vi "LR-Spikes.vi"(5 "Test characteristics":T2, 7 "Spike detection settings":cluster{"Treshold [%]":i32}={"Treshold [%]"=10}, 8 "error in (no error)":errorcluster, 9 "Power in":dbl[](array[numeric]), 11 "Results in":T1) -> (0 "error out":errorcluster, 1 "Power":dbl[](array[numeric]), 3 "Results":T1, 4 "Valid?":bool)   [LabVIEW 2013, in "MaterialCharacterization.lvlib" / "MC-LaserResponse.lvclass"]
doc: "Use this template to build a VI to use as a subVI."
uses:
  MC-LaserResponse.lvclass
  Test-characteristics.ctl
  Detectors.ctl
  Test-results.ctl
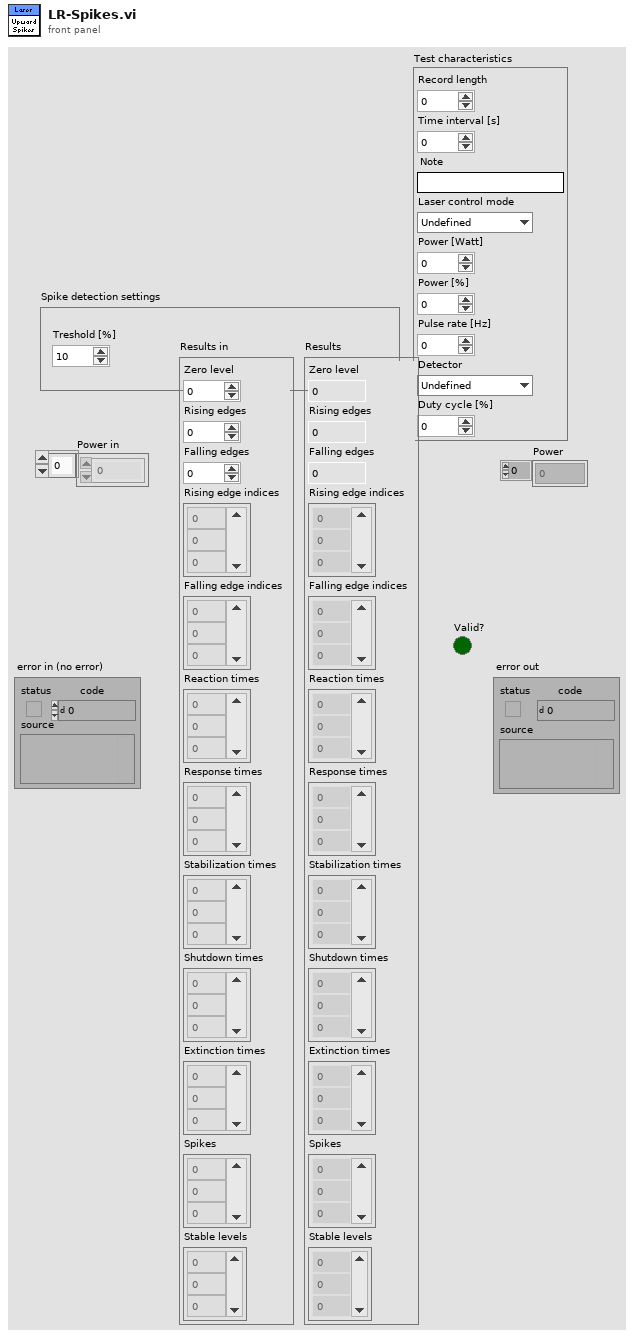
[diagram p1: front panel]
types:
  T1 = typedef "MaterialCharacterization.lvlib/MC-LaserResponse.lvclass/Test-results.ctl" = cluster{"Zero level":dbl, "Rising edges":i32, "Falling edges":i32, "Rising edge indices":dbl[], "Falling edge indices":dbl[], "Reaction times":dbl[], "Response times":dbl[], "Stabilization times":dbl[], "Shutdown times":dbl[], "Extinction times":dbl[], "Spikes":i32[], "Stable levels":dbl[]}
  T2 = typedef "MaterialCharacterization.lvlib/MC-LaserResponse.lvclass/Test-characteristics.ctl" = cluster{"Record length":i32, "Time interval [s]":dbl, "Note":string, "Laser control mode":enum16{"Undefined", "Modulation (digital)", "Power variation (analog)"}, "Power [Watt]":dbl, "Power [%]":dbl, "Pulse rate [Hz]":dbl, "Detector":T3, "Duty cycle [%]":dbl}
  T3 = typedef "MaterialCharacterization.lvlib/MC-LaserResponse.lvclass/Detectors.ctl" = enum16{"Undefined", "DET10A", "DET10A - 2kOhm ", "PDA36A - 0dB"}
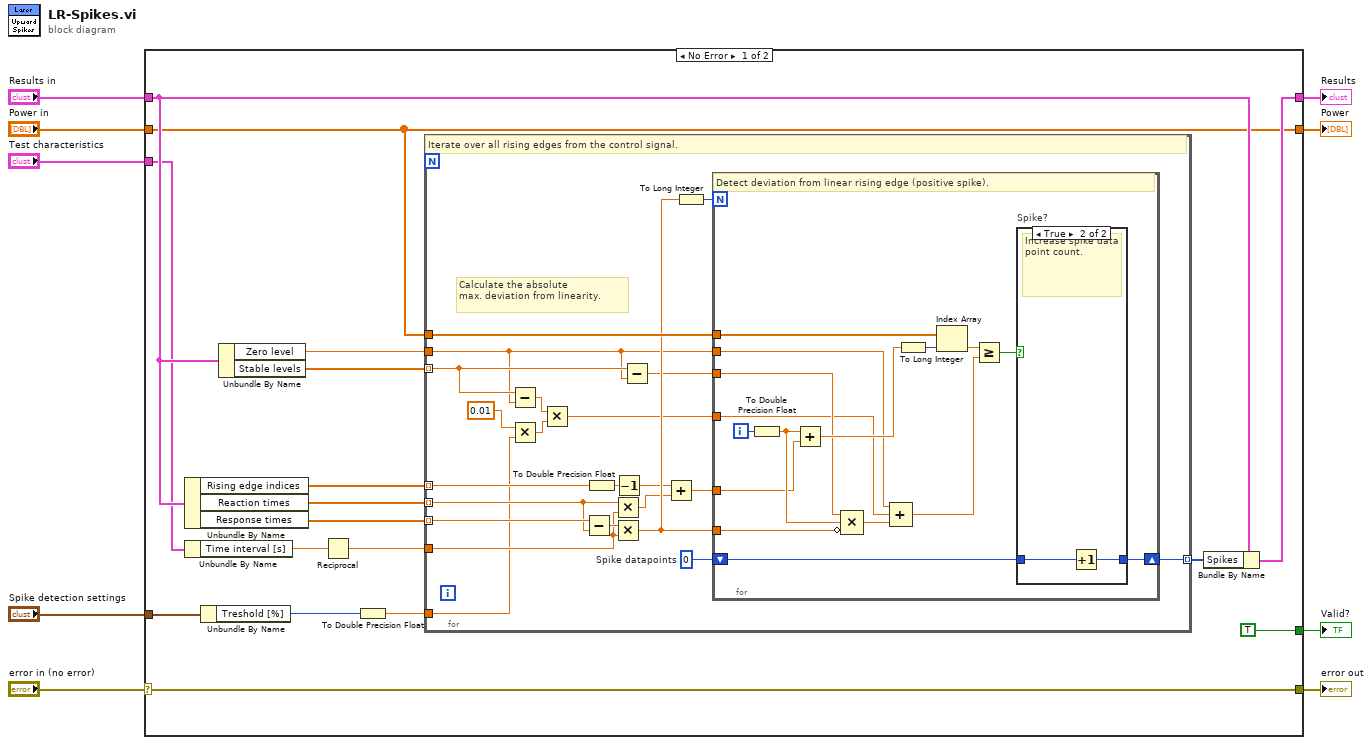
[diagram p0: block diagram]
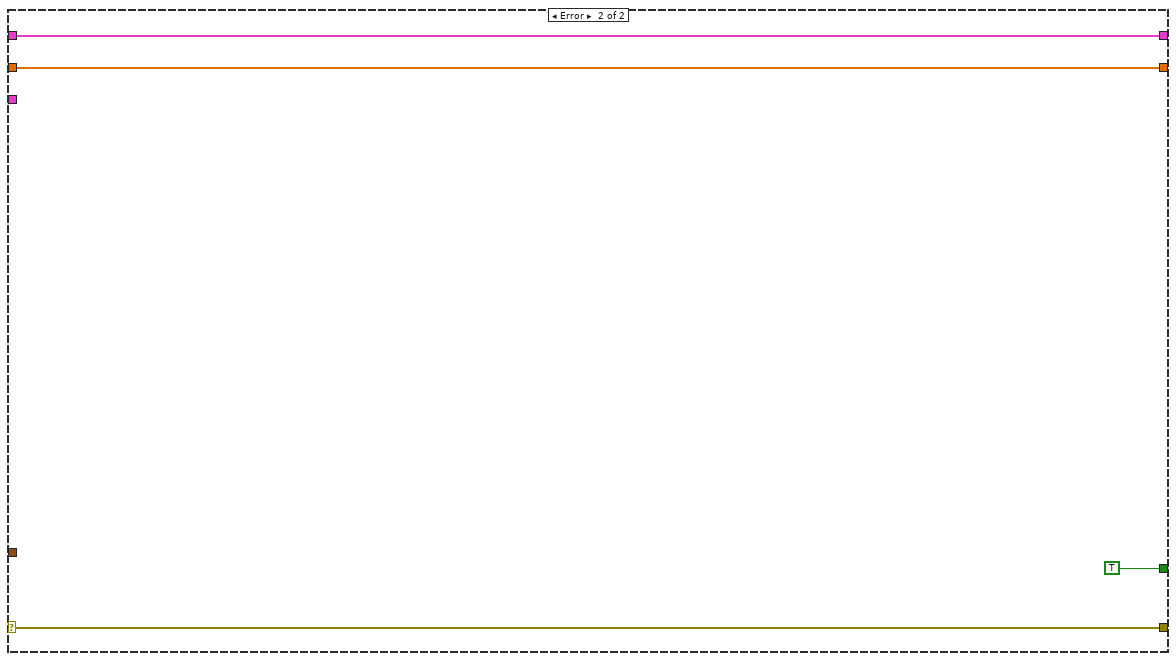
[diagram p3: hidden frame]
diagram:
  n1 = case shown="No Error" "error in (no error)" {
    selector: "error in (no error)" -> [w25 w71]
    tunnel: [w25 w71] -> w1
    tunnel: "Results in" -> [w23 w70]
    tunnel: "Spike detection settings" -> [w26 _]
    tunnel: [TRUE TRUE] -> w4
    tunnel: [w24 w70] -> w3
    tunnel: "Power in" -> [w14 w68]
    tunnel: "Test characteristics" -> [w15 _]
    tunnel: [w14 w68] -> w2
    frame No Error {
      n2 = Unbundle By Name(w23) -> ("Rising edge indices"=w22:dbl[], "Reaction times"=w21:dbl[], "Response times"=w20:dbl[])
      n3 = Unbundle By Name(w15) -> ("Time interval [s]"=w19:dbl)
      n4 = Unbundle By Name(w26) -> ("Treshold [%]"=w11:i32)
      n5 = Unbundle By Name(w23) -> ("Zero level"=w13:dbl, "Stable levels"=w12:dbl[])
      n6 = Reciprocal(x=w19) -> (1/x=w18:dbl)
      n7 = To Double Precision Float(number=w11) -> (double precision float=w10:dbl)
      n8 = for {
        tunnel: w14 -> [w48]
        tunnel: w22 -> [w47] mode=indexing
        tunnel: w21 -> [w43] mode=indexing
        tunnel: w20 -> [w46] mode=indexing
        tunnel: w18 -> [w44]
        tunnel: [w35] -> w17 mode=indexing
        tunnel: w13 -> [w27]
        tunnel: w12 -> [w31] mode=indexing
        tunnel: w10 -> [w30]
        w36 = 0  # Spike datapoints
        # "Calculate the absolute\nmax. deviation from linearity."
        # "Iterate over all rising edges from the control signal."
        n9 = Subtract(x=w31, y=w27) -> (x-y=w32:dbl)
        n10 = Multiply(x=0.01, y=w30) -> (x*y=w33:dbl)
        n11 = Multiply(x=w32, y=w33) -> (x*y=w29:dbl)
        n12 = Subtract(x=w46, y=w43) -> (x-y=w45:dbl)
        n13 = To Double Precision Float(number=w47) -> (double precision float=w42:dbl)
        n14 = Multiply(x=w43, y=w44) -> (x*y=w39:dbl)
        n15 = Multiply(x=w45, y=w44) -> (x*y=w41:dbl)
        n16 = Decrement(x=w42) -> (x-1=w38:dbl)
        n17 = Subtract(x=w31, y=w27) -> (x-y=w28:dbl)
        n18 = Add(x=w38, y=w39) -> (x+y=w37:dbl)
        n19 = To Long Integer(number=w41) -> (32bit integer=w40:i32)
        n20 = for {
          N: w40 -> [_]
          tunnel: w48 -> [w64]
          tunnel: w29 -> [w56]
          tunnel: w41 -> [w60]
          tunnel: w28 -> [w61]
          tunnel: w27 -> [w53]
          tunnel: w37 -> [w58]
          shift-right: [w49] -> w35
          shift-left: w36 -> [w50]
          i -> [w62]
          # "Detect deviation from linear rising edge (positive spike)."
          n21 = To Double Precision Float(number=w62) -> (double precision float=w59:dbl)
          n22 = Add(x=w59, y=w58) -> (x+y=w63:dbl)
          n23 = Compound Arithmetic op=MULTIPLY(w61, w59, invert w60) -> (w57:dbl)
          n24 = Compound Arithmetic op=ADD(w53, w56, w57) -> (w52:dbl)
          n25 = To Long Integer(number=w63) -> (32bit integer=w54:i32)
          n26 = Index Array(array=w64, index=w54) -> (element=w55:dbl)
          n27 = Greater Or Equal?(x=w55, y=w52) -> (x >= y?=w51:bool)
          n28 = case "Spike?" shown="True" w51 {
            tunnel: w50 -> [w65 w67]
            tunnel: [w65 w66] -> w49
            frame False {
              # "Do nothing."
            }
            frame True {
              # "Increase spike data point count."
              n29 = Increment(x=w67) -> (x+1=w66:i32)
            }
          }
        }
      }
      n30 = Bundle By Name(cluster=w23, "Spikes"=w17) -> (w24:T1)
    }
    frame Error {
    }
  }
  "Valid?" <- w4
  "Results" <- w3
  "Power" <- w2
  "error out" <- w1
